vi "MultiVoltageSource.vi"() -> ()   [LabVIEW 2020]
uses:
  <vilib>/Instr/_visa.llb/VISA Configure Serial Port (Instr).vi
panel:
  in  "Alias Ch 7":string
  in  "Alias Ch 6":string
  in  "Alias Ch 5":string
  in  "Alias Ch 4":string
  in  "Alias Ch 3":string
  in  "Alias Ch 2":string
  in  "Alias Ch 1":string
  in  "Source Alias":string
  in  "Reset Button":bool
  in  "Channel 7":dbl=0.2 min=0.2 max=10.2 step=0.1 format="%_2f"
  in  "Channel 6":dbl=0.2 min=0.2 max=10.2 step=0.1 format="%_2f"
  in  "Channel 5":dbl=0.2 min=0.2 max=10.2 step=0.1 format="%_2f"
  in  "Channel 4":dbl=0.2 min=0.2 max=10.2 step=0.1 format="%_2f"
  in  "Channel 3":dbl=0.2 min=0.2 max=10.2 step=0.1 format="%_2f"
  in  "Channel 2":dbl=0.2 min=0.2 max=10.2 step=0.1 format="%_2f"
  in  "Channel 1":dbl=0.2 min=0.2 max=10.2 step=0.1 format="%_2f"
  in  "STOP":bool
  in  "MultiVoltageSource USB Port":refnum<visa-resource-name>
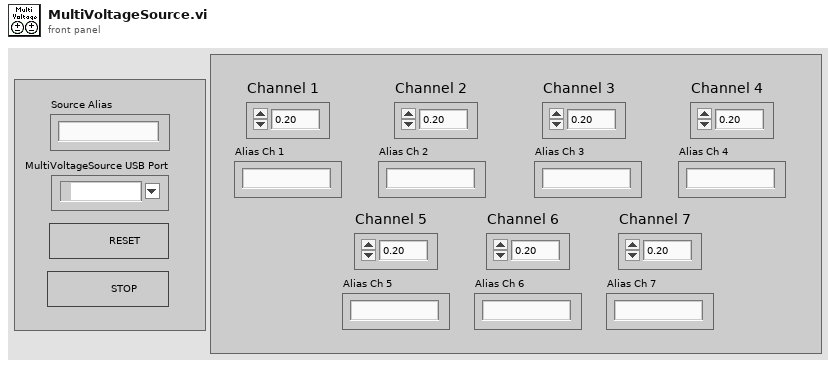
[diagram p1: front panel]
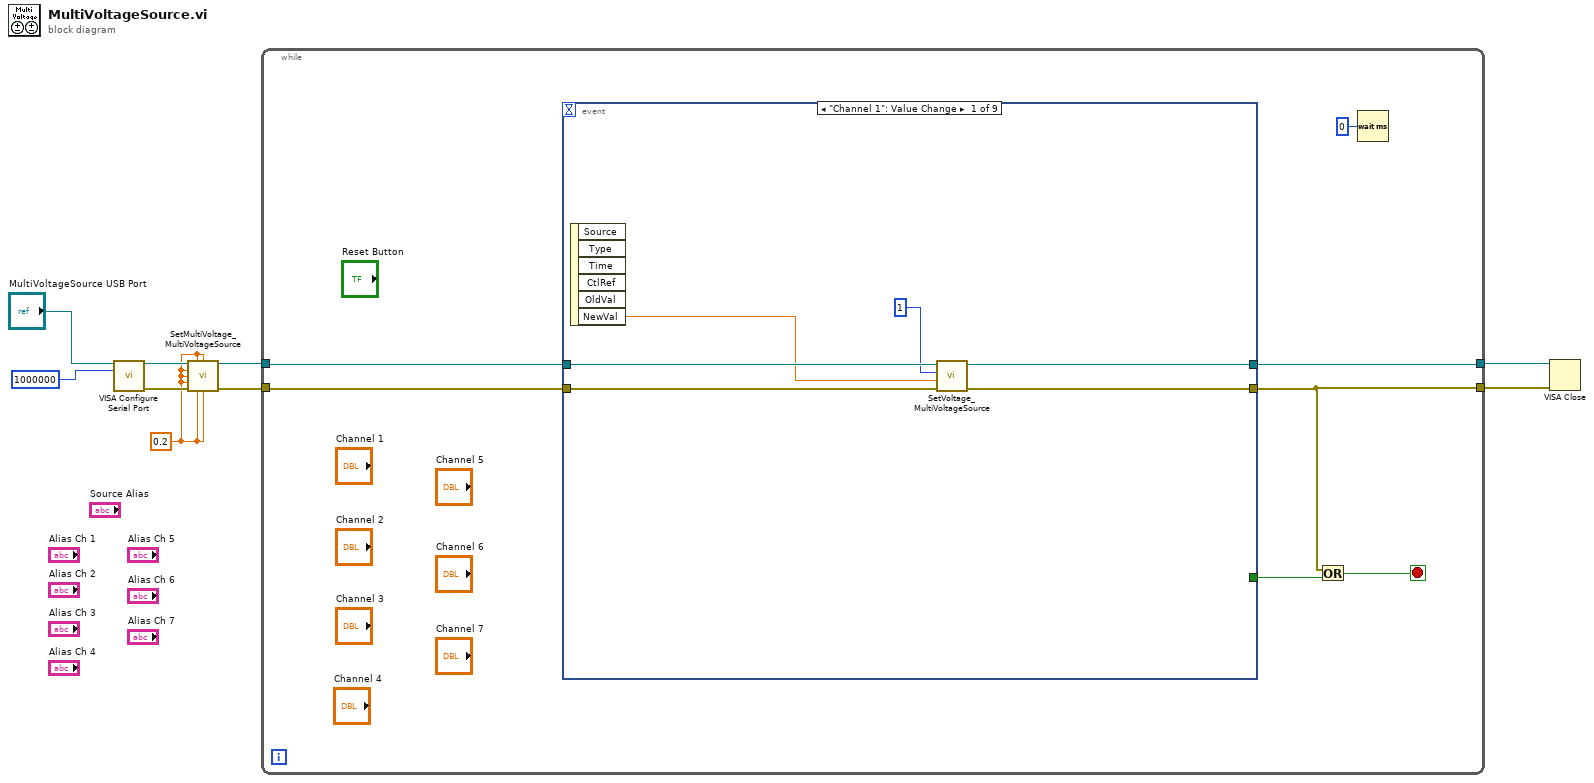
[diagram p0: block diagram]
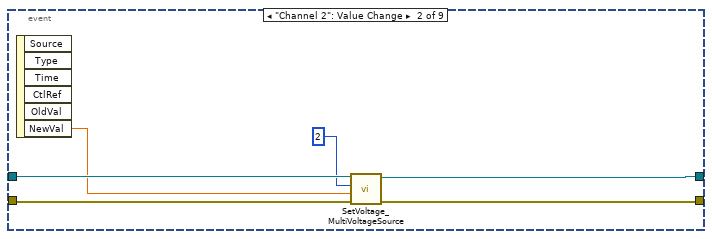
[diagram p2: hidden frame]
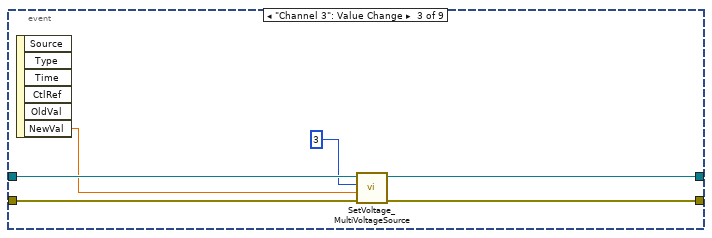
[diagram p3: hidden frame]
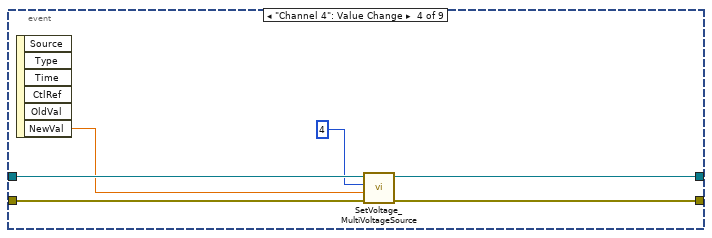
[diagram p4: hidden frame]
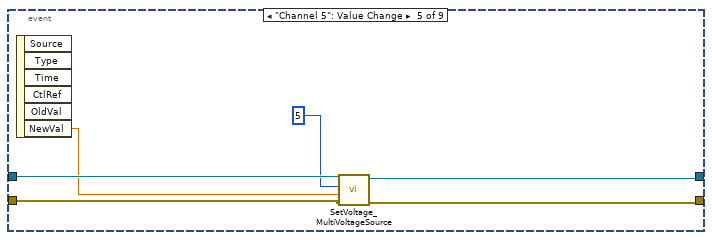
[diagram p5: hidden frame]
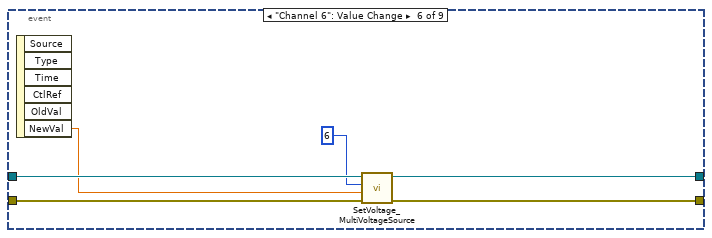
[diagram p6: hidden frame]
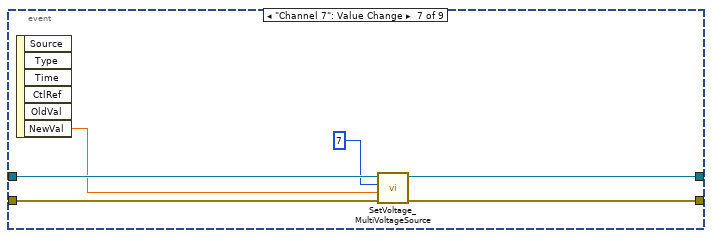
[diagram p7: hidden frame]
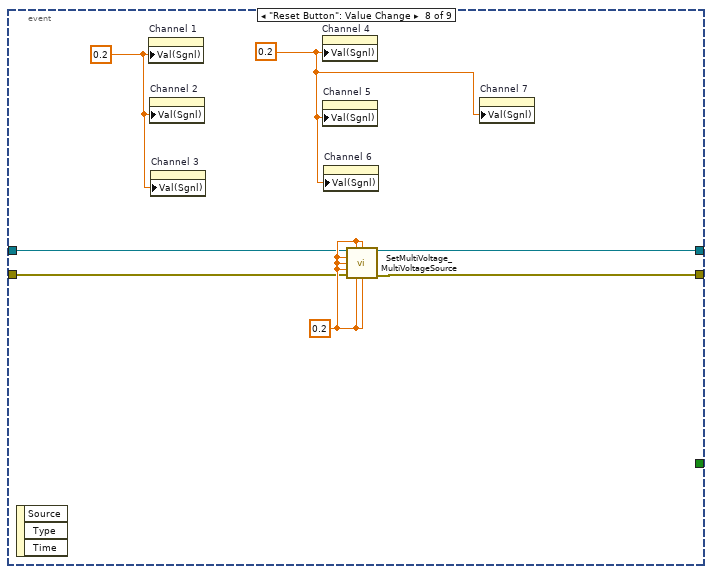
[diagram p8: hidden frame]
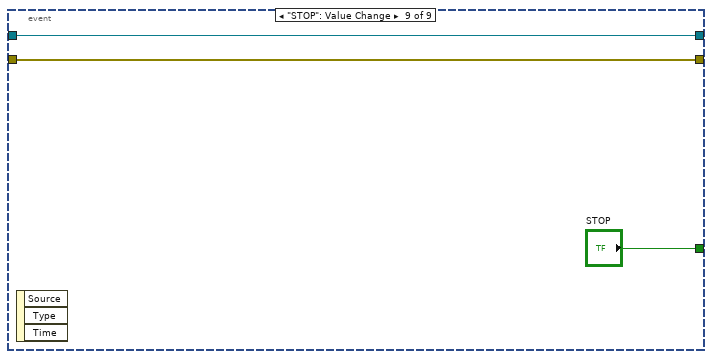
[diagram p9: hidden frame]
diagram:
  w1 = 0.2 ("Channel Value")
  n1 = call-poly "VISA Configure Serial Port"("VISA resource name"="MultiVoltageSource USB Port", "baud rate (9600)"=u32 1000000) -> ("VISA resource name out"=w3:refnum<visa-resource-name>, "error out"=w2:errorcluster)  [unwired: 12 in]
  n2 = call "SetMultiVoltage_MultiVoltageSource.vi"("VISA Refnum in"=w3, "Channel Value 6"=w1, "Channel Value 7"=w1, "Channel Value 5"=w1, "Channel Value 4"=w1, "Channel Value 3"=w1, "error in (no error)"=w2, "Channel Value 2"=w1, "Channel Value"=w1) -> ("VISA Refnum out"=w5:refnum<visa-resource-name>, "error out"=w4:errorcluster)  [unwired: 5 in]
  n3 = while {
    tunnel: w5 -> [w16]
    tunnel: w4 -> [w14]
    tunnel: [w12] -> w8
    tunnel: [w15] -> w7
    stop <- w11 stop-if-true
    n4 = event shown="[0] \"Channel 1\": Value Change" {
      selector: _ -> [_ _ _ _ _ _ _ _ _]
      dyn-events: _ -> [_ _ _ _ _ _ _ _ _]
      timeout: _ -> [_ _ _ _ _ _ _ _ _]
      tunnel: w16 -> [w22 w28 w34 w40 w46 w52 w58 w64 w67]
      tunnel: [w19 w26 w31 w37 w43 w50 w56 w61 w67] -> w15
      tunnel: w14 -> [w21 w27 w33 w39 w45 w51 w57 w63 w66]
      tunnel: [w20 w25 w32 w38 w44 w49 w55 w62 w66] -> w12
      tunnel: [_ _ _ _ _ _ _ _ "STOP"] -> w13
      event "Channel 1": Value Change {
        n5 = event-data() -> ("NewVal"=w17:dbl)  [unwired: 1 in, 5 out]
        n6 = call "SetVoltage_MultiVoltageSource.vi"("error in (no error)"=w21, "Channel Value"=w17, "Channel"=1, "VISA Refnum in"=w22) -> ("error out"=w20:errorcluster, "VISA Refnum out"=w19:refnum<visa-resource-name>)  [unwired: 6 in]
      }
      event "Channel 2": Value Change {
        n7 = event-data() -> ("NewVal"=w23:dbl)  [unwired: 1 in, 5 out]
        n8 = call "SetVoltage_MultiVoltageSource.vi"("error in (no error)"=w27, "Channel Value"=w23, "Channel"=2, "VISA Refnum in"=w28) -> ("error out"=w25:errorcluster, "VISA Refnum out"=w26:refnum<visa-resource-name>)  [unwired: 6 in]
      }
      event "Channel 3": Value Change {
        n9 = event-data() -> ("NewVal"=w29:dbl)  [unwired: 1 in, 5 out]
        n10 = call "SetVoltage_MultiVoltageSource.vi"("error in (no error)"=w33, "Channel Value"=w29, "Channel"=3, "VISA Refnum in"=w34) -> ("error out"=w32:errorcluster, "VISA Refnum out"=w31:refnum<visa-resource-name>)  [unwired: 6 in]
      }
      event "Channel 4": Value Change {
        n11 = event-data() -> ("NewVal"=w35:dbl)  [unwired: 1 in, 5 out]
        n12 = call "SetVoltage_MultiVoltageSource.vi"("error in (no error)"=w39, "Channel Value"=w35, "Channel"=4, "VISA Refnum in"=w40) -> ("error out"=w38:errorcluster, "VISA Refnum out"=w37:refnum<visa-resource-name>)  [unwired: 6 in]
      }
      event "Channel 5": Value Change {
        n13 = event-data() -> ("NewVal"=w41:dbl)  [unwired: 1 in, 5 out]
        n14 = call "SetVoltage_MultiVoltageSource.vi"("error in (no error)"=w45, "Channel Value"=w41, "Channel"=5, "VISA Refnum in"=w46) -> ("error out"=w44:errorcluster, "VISA Refnum out"=w43:refnum<visa-resource-name>)  [unwired: 6 in]
      }
      event "Channel 6": Value Change {
        n15 = event-data() -> ("NewVal"=w47:dbl)  [unwired: 1 in, 5 out]
        n16 = call "SetVoltage_MultiVoltageSource.vi"("error in (no error)"=w51, "Channel Value"=w47, "Channel"=6, "VISA Refnum in"=w52) -> ("error out"=w49:errorcluster, "VISA Refnum out"=w50:refnum<visa-resource-name>)  [unwired: 6 in]
      }
      event "Channel 7": Value Change {
        n17 = event-data() -> ("NewVal"=w53:dbl)  [unwired: 1 in, 5 out]
        n18 = call "SetVoltage_MultiVoltageSource.vi"("error in (no error)"=w57, "Channel Value"=w53, "Channel"=7, "VISA Refnum in"=w58) -> ("error out"=w55:errorcluster, "VISA Refnum out"=w56:refnum<visa-resource-name>)  [unwired: 6 in]
      }
      event "Reset Button": Value Change {
        w59 = 0.2 ("Channel Value")
        w60 = 0.2 ("Channel Value")
        w65 = 0.2 ("Channel Value")
        n19 = event-data() -> ()  [unwired: 1 in, 3 out]
        n20 = property on="Channel 1" class="DigNum (strict)"("Val(Sgnl)"=w60) -> ()  [unwired: 2 in, 2 out]
        n21 = property on="Channel 2" class="DigNum (strict)"("Val(Sgnl)"=w60) -> ()  [unwired: 2 in, 2 out]
        n22 = property on="Channel 3" class="DigNum (strict)"("Val(Sgnl)"=w60) -> ()  [unwired: 2 in, 2 out]
        n23 = property on="Channel 4" class="DigNum (strict)"("Val(Sgnl)"=w59) -> ()  [unwired: 2 in, 2 out]
        n24 = property on="Channel 5" class="DigNum (strict)"("Val(Sgnl)"=w59) -> ()  [unwired: 2 in, 2 out]
        n25 = property on="Channel 6" class="DigNum (strict)"("Val(Sgnl)"=w59) -> ()  [unwired: 2 in, 2 out]
        n26 = call "SetMultiVoltage_MultiVoltageSource.vi"("VISA Refnum in"=w64, "Channel Value 6"=w65, "Channel Value 7"=w65, "Channel Value 5"=w65, "Channel Value 4"=w65, "Channel Value 3"=w65, "error in (no error)"=w63, "Channel Value 2"=w65, "Channel Value"=w65) -> ("VISA Refnum out"=w61:refnum<visa-resource-name>, "error out"=w62:errorcluster)  [unwired: 5 in]
        n27 = property on="Channel 7" class="DigNum (strict)"("Val(Sgnl)"=w59) -> ()  [unwired: 2 in, 2 out]
      }
      event "STOP": Value Change {
        n28 = event-data() -> ()  [unwired: 1 in, 3 out]
      }
    }
    n29 = Or(x=w12, y=w13) -> (x .or. y?=w11:bool)
    n30 = Wait (ms)(milliseconds to wait=u32 0) -> ()  [unwired: 1 out]
  }
  n31 = VISA Close(VISA resource name=w7, error in (no error)=w8) -> ()  [unwired: 1 out]
